vi "SetupDMA.vi"(1 "pixel":u32=2400, 2 "nos":u32=1) -> (0 "Data Values":u16[][](graph))   [LabVIEW 2015]
uses:
  ESLSCDLL.dll
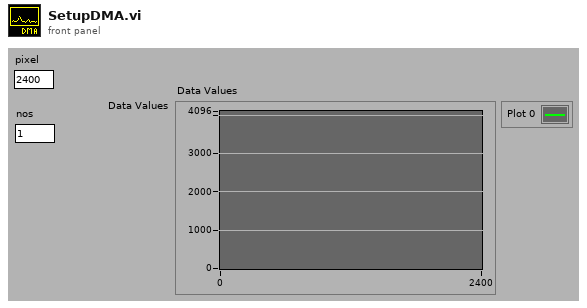
[diagram p1: front panel]
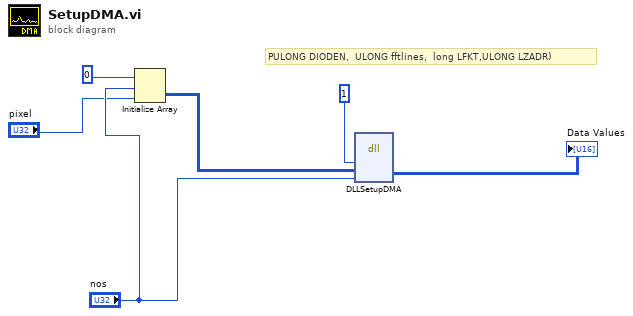
[diagram p0: block diagram]
diagram:
  # "PULONG DIODEN, \tULONG fftlines,  long LFKT,ULONG LZADR)"
  n1 = Initialize Array(u32 0, "nos", "pixel") -> (w4:u32[][])
  n2 = dll-call lib="C:/ENTW/PCIE/64bit/lv64/1cam/board.vis/ESLSCDLL.dll" fn="DLLSetupDMA" ("lwlscdll.dll:DLLReadFFLoop")("drv"=u32 1, "dioden"=w4, "nos"="nos") -> ("dioden"=→"Data Values":u16[][])  [unwired: 6 in, 2 out]
